vi "Pre Launch Init.vi"(11 "Instrument Handler in":refnum<class "Instrument Handler.lvclass">) -> (0 "error out":errorcluster, 3 "Instrument Handler out":refnum<class "Instrument Handler.lvclass">)   [LabVIEW 2020, in "Instrument Handler.lvlib" / "Instrument Handler.lvclass"]
doc: "(<B>Filename</B>: Actor Framework.lvlib:Actor.lvclass:Pre Launch Init.vi)\n\nDefines behavior that occurs after the Launch Nested Actor method is invoked but before the actor's Actor Core method begins running.\n\nThis implementation obtains the Aquirer Lock Semaphore for use with the Multi Instrument Handler actors. The launch is aborted if an Instrument Handler is already running."
uses:
  Instrument Handler.lvclass
  C:/Current projects/WS/PPL/HDH.Actor Framework.Core.Actor.lvlibp/1abvi3w/vi.lib/ActorFramework/Actor/Actor.lvclass
  Instrument Handler.lvclass/Instrument Handler.ctl
  Enqueuer Global.vi
  PPL/HDH.Actor Framework.Core.Actor.lvlibp/1abvi3w/vi.lib/ActorFramework/Actor/Actor.lvclass
  PPL/HDH.Actor Framework.Core.Actor.lvlibp/1abvi3w/vi.lib/ActorFramework/Message Enqueuer/Message Enqueuer.lvclass
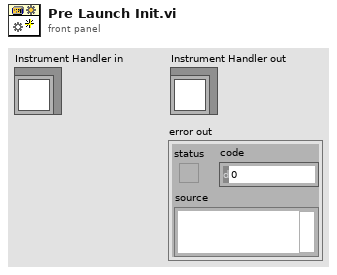
[diagram p1: front panel]
types:
  T1 = typedef "Semaphore RefNum" = refnum<k1>
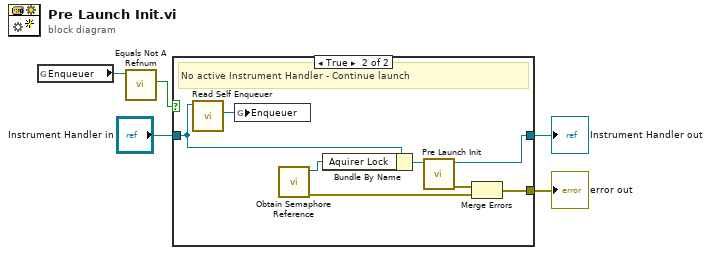
[diagram p0: block diagram]
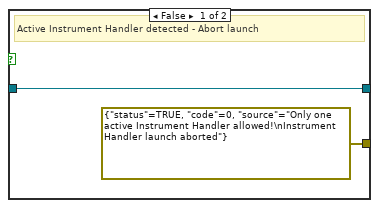
[diagram p2: hidden frame]
diagram:
  n1 = global read "Enqueuer Global.vi" "Enqueuer"() -> (w2:refnum<class "Message Enqueuer.lvclass">)
  n2 = call "Equals Not A Refnum.vi"("Message Enqueuer"=w2) -> ("Not a refnum?"=w1:bool)  [unwired: 10 in]
  n3 = case shown="True" w1 {
    tunnel: [w7 w14] -> w5
    tunnel: "Instrument Handler in" -> [w7 w9]
    tunnel: [errorcluster {"status"=TRUE, "code"=0, "source"="Only one active Instrument Handler allowed!\nInstrument Handler launch aborted"} ("error IO") w11] -> w3
    frame False {
      # "Active Instrument Handler detected - Abort launch"
    }
    frame True {
      # "No active Instrument Handler - Continue launch"
      n4 = call "Read Self Enqueuer.vi"("Actor"=w9) -> ("Self Enqueuer"=w8:refnum<class "Message Enqueuer.lvclass">)  [unwired: 10 in]
      n5 = global write "Enqueuer Global.vi" "Enqueuer"(w8) -> ()
      n6 = call <vilib>:"Obtain Semaphore Reference.vi"() -> ("error out"=w10:errorcluster, "semaphore"=w12:T1)  [unwired: 5 in, 1 out]
      n7 = Bundle By Name(cluster=w9, "Aquirer Lock"=w12) -> (w13:refnum<class "Instrument Handler.lvclass">)
      n8 = call-parent "Pre Launch Init.vi"("Actor in"=w13) -> ("error out"=w15:errorcluster, "Actor out"=w14:refnum<class "Instrument Handler.lvclass">)  [unwired: 9 in]
      n9 = Merge Errors(w15, w10) -> (w11:errorcluster)
    }
  }
  "error out" <- w3
  "Instrument Handler out" <- w5
